vi "ROS_publisher.vi"() -> ()   [LabVIEW 2017]
uses:
  <vilib>/Tufts CEEO ROS for LabVIEW Software/ROS/Code/Console/Servers/ServerSubs/TopicDef.ctl
  <vilib>/Tufts CEEO ROS for LabVIEW Software/ROS/Code/SubVIs/_ROSDirection.ctl
  <vilib>/Tufts CEEO ROS for LabVIEW Software/ROS/MessageBuilding/std_msgs/subs/float32Scalar.vi
panel:
  in  "Numeric":sgl
  out "error out":errorcluster
  in  "stop":bool
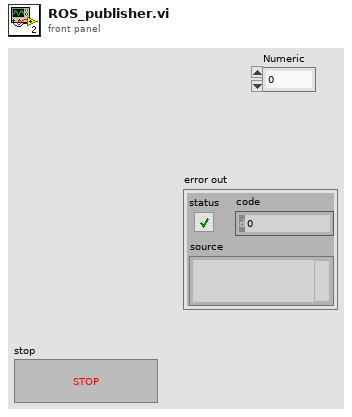
[diagram p1: front panel]
types:
  T1 = typedef "TopicDef.ctl" = cluster{"Topic":string, "Type":string, "Action":T2, "Update (ms)":u16, "queue size":u16}
  T2 = typedef "_ROSDirection.ctl" = enum16{"Node", "Publisher", "Subscriber", "ServiceClient", "ServiceProvider"}
  T3 = typedef "_ROSControl.ctl" = cluster{"topic port":u16, "Node":string, "topic":string, "type":string, "node port":u16, "error ":errorcluster, "Direction":T2, "Update (ms)":u16, "FIFO size":u16}
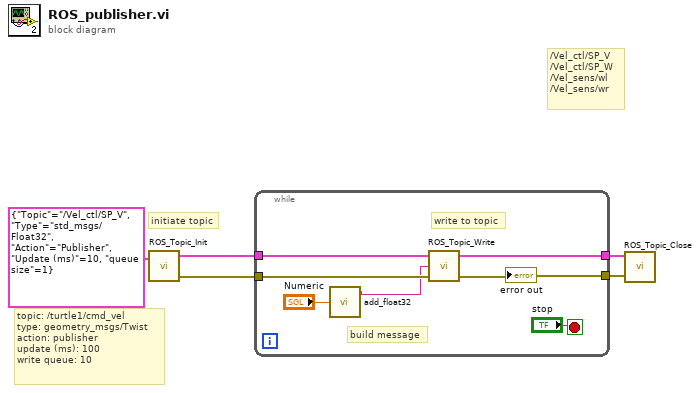
[diagram p0: block diagram]
diagram:
  # "initiate topic"
  # "topic: /turtle1/cmd_vel\ntype: geometry_msgs/Twist\naction: publisher\nupdate (ms): 100\nwrite queue: 10"
  # "/Vel_ctl/SP_V\n/Vel_ctl/SP_W\n/Vel_sens/wl\n/Vel_sens/wr"
  n1 = call <vilib>:"ROS_Topic_Init.vi"("Definitions"=T1 {"Topic"="/Vel_ctl/SP_V", "Type"="std_msgs/Float32", "Action"=enum."Publisher", "Update (ms)"=10, "queue size"=1}) -> ("ROS out"=w4:T3, "error out"=w3:errorcluster)  [unwired: 2 in]
  n2 = while {
    tunnel: w4 -> [w12]
    tunnel: w3 -> [w11]
    tunnel: [w9] -> w2
    tunnel: [w8] -> w1
    stop <- "stop" stop-if-true
    # "build message"
    # "write to topic"
    n3 = call-poly <vilib>:"add_float32.vi"("Numeric"="Numeric") -> ("msg out"=w7:string)  [unwired: 4 in]
    n4 = call <vilib>:"ROS_Topic_Write.vi"("error in (no error)"=w11, "Msg in"=w7, "ROS in"=w12) -> ("error out"=w8:errorcluster, "ROS out"=w9:T3)  [unwired: 1 in]
    "error out" <- w8
  }
  n5 = call <vilib>:"ROS_Topic_Close.vi"("error in"=w1, "ROS in"=w2) -> ()  [unwired: 2 in, 1 out]
